vi "2_ExportDatatoExcel.vi"(8 "error in (no error)":errorcluster, 10 "Waveform Graph":waveform(dbl)[](graph), 11 "file path (IN)":path) -> (0 "error out":errorcluster, 3 "file path (OUT)":path)   [LabVIEW 2020]
uses:
  <vilib>/Utility/file.llb/Write Delimited Spreadsheet (string).vi
panel:
  out "Ch3 : Y":dbl[](array[numeric])
  out "Ch3 : appended array":string[](array[string])
  out "Ch2 : Y":dbl[](array[numeric])
  out "Ch2 : appended array":string[](array[string])
  out "Ch1 : appended array":string[](array[string])
  out "Ch1 : Y":dbl[](array[numeric])
  out "dt":dbl
  out "Spread Sheet Display":string[][](array[string])
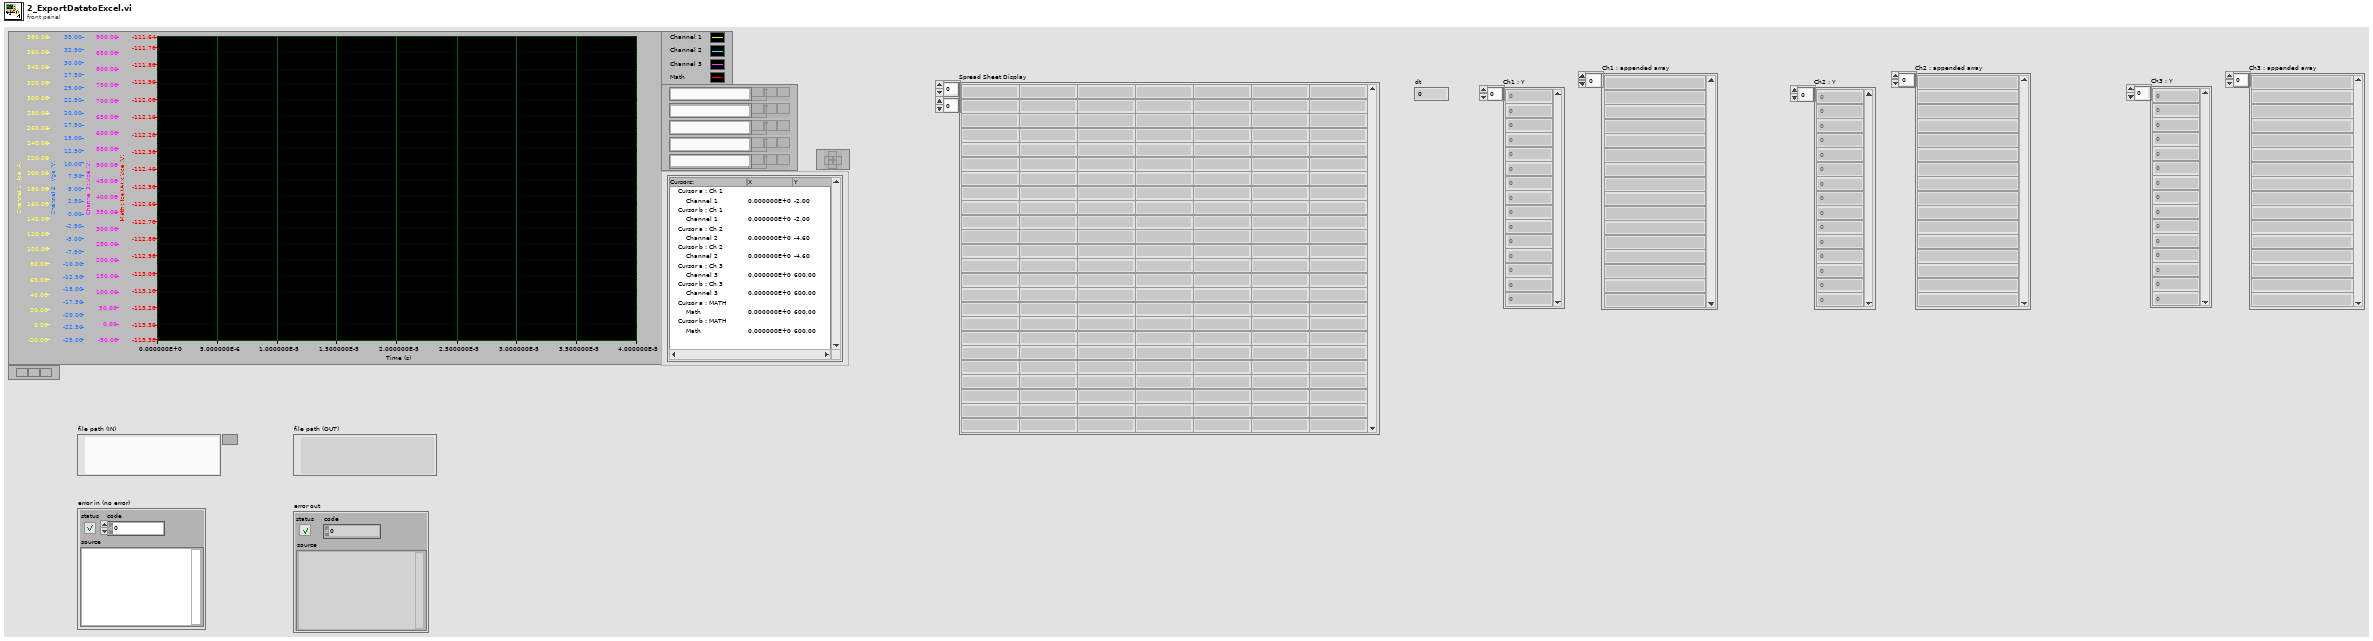
[diagram p1: front panel]
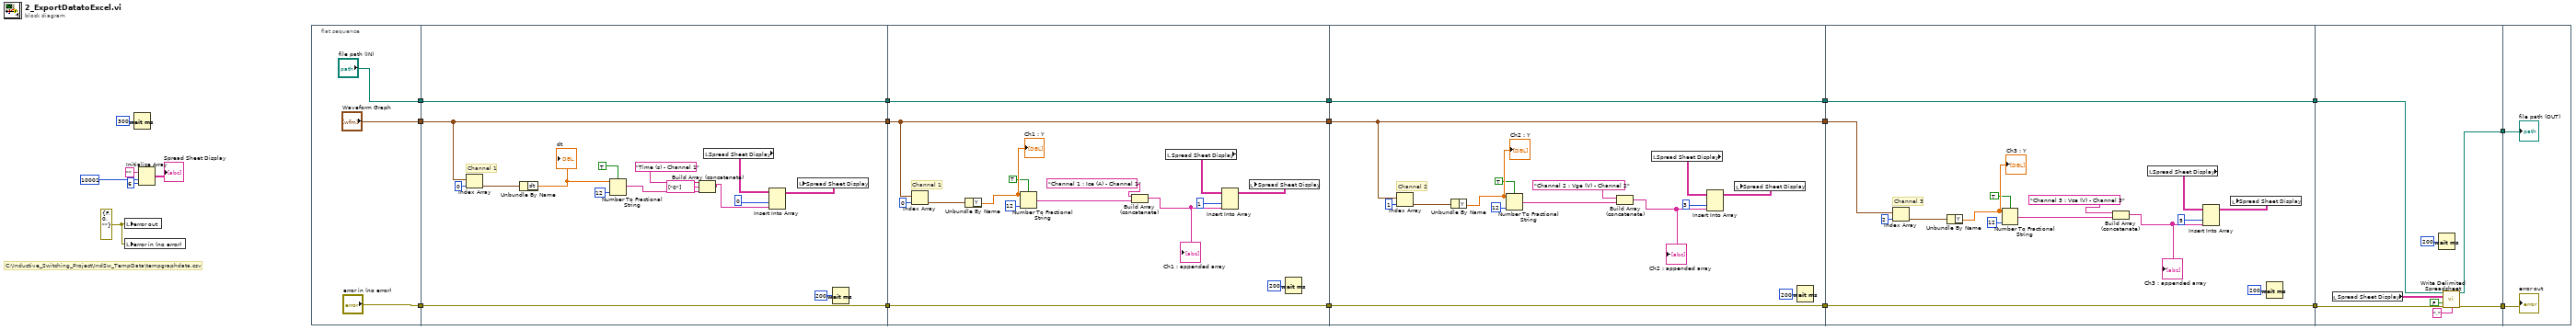
[diagram p0: block diagram]
diagram:
  w7 = errorcluster {"status"=FALSE, "code"=0, "source"=""} ("error out")
  # "C:\\Inductive_Switching_Project\\IndSw_TempData\\tempgraphdata.csv"
  n1 = local write "error out"(w7) -> ()
  n2 = local write "error in (no error)"(w7) -> ()
  n3 = Wait (ms)(milliseconds to wait=u32 300) -> ()  [unwired: 1 out]
  n4 = Initialize Array("", 10001 ("dimension size"), 6 ("dimension size")) -> (→"Spread Sheet Display":string[][])
  n5 = flat-sequence {
    tunnel: ["Waveform Graph"] -> w13
    tunnel: ["error in (no error)"] -> w9
    tunnel: ["file path (IN)"] -> w2
    tunnel: [w29] -> w17
    tunnel: w13 -> [w29]
    tunnel: w9 -> [w28]
    tunnel: [w28] -> w8
    tunnel: [w26] -> w3
    tunnel: w2 -> [w26]
    tunnel: w17 -> [w45]
    tunnel: [w45] -> w16
    tunnel: [w44] -> w10
    tunnel: w8 -> [w44]
    tunnel: [w42] -> w4
    tunnel: w3 -> [w42]
    tunnel: w16 -> [w60]
    tunnel: [w60] -> w15
    tunnel: [w59] -> w11
    tunnel: w10 -> [w59]
    tunnel: [w57] -> w5
    tunnel: w4 -> [w57]
    tunnel: w15 -> [w75]
    tunnel: [w74] -> w12
    tunnel: w11 -> [w74]
    tunnel: [w72] -> w6
    tunnel: w5 -> [w72]
    tunnel: [w91] -> w14
    tunnel: w12 -> [w90]
    tunnel: w6 -> [w88]
    tunnel: [w87] -> w1
    tunnel: w14 -> [w96]
    tunnel: w1 -> [w95]
    frame #0 {
    }
    frame #1 {
      # "Channel 1"
      n6 = Index Array(array=w29, index=0) -> (element=w40:waveform(dbl))
      n7 = Unbundle By Name(w40) -> ("dt"=w38:dbl)
      "dt" <- w38
      n8 = Number To Fractional String(use system decimal point (T)=TRUE, number=w38, precision (6)=i16 12) -> (F-format string=w33:string)  [unwired: 1 in]
      n9 = Build Array (concatenate)("Time (s) - Channel 1", string[] ["0"] ("array"), w33) -> (w32:string[])
      n10 = local read "Spread Sheet Display"() -> (w37:string[][])
      n11 = Insert Into Array(array=w37, index (col)=0 ("disabled index (col)"), new element=w32) -> (w41:string[][])  [unwired: 1 in]
      n12 = local write "Spread Sheet Display"(w41) -> ()
      n13 = Wait (ms)(milliseconds to wait=u32 200) -> ()  [unwired: 1 out]
    }
    frame #2 {
      # "Channel 1"
      n14 = Index Array(array=w45, index=0) -> (element=w52:waveform(dbl))
      n15 = Unbundle By Name(w52) -> ("Y"=w53:dbl[])
      "Ch1 : Y" <- w53
      n16 = Number To Fractional String(use system decimal point (T)=TRUE, number=w53, precision (6)=i16 12) -> (F-format string=w55:string[])  [unwired: 1 in]
      n17 = Build Array (concatenate)("Channel 1 : Ice (A) - Channel 1", w55) -> (w56:string[])
      "Ch1 : appended array" <- w56
      n18 = local read "Spread Sheet Display"() -> (w54:string[][])
      n19 = Insert Into Array(array=w54, index (col)=1 ("disabled index (col)"), new element=w56) -> (w51:string[][])  [unwired: 1 in]
      n20 = local write "Spread Sheet Display"(w51) -> ()
      n21 = Wait (ms)(milliseconds to wait=u32 200) -> ()  [unwired: 1 out]
    }
    frame #3 {
      # "Channel 2"
      n22 = Index Array(array=w60, index=1) -> (element=w71:waveform(dbl))
      n23 = Unbundle By Name(w71) -> ("Y"=w70:dbl[])
      "Ch2 : Y" <- w70
      n24 = Number To Fractional String(use system decimal point (T)=TRUE, number=w70, precision (6)=i16 12) -> (F-format string=w68:string[])  [unwired: 1 in]
      n25 = Build Array (concatenate)("Channel 2 : Vge (V) - Channel 2", w68) -> (w67:string[])
      "Ch2 : appended array" <- w67
      n26 = local read "Spread Sheet Display"() -> (w69:string[][])
      n27 = Insert Into Array(array=w69, index (col)=3 ("disabled index (col)"), new element=w67) -> (w66:string[][])  [unwired: 1 in]
      n28 = local write "Spread Sheet Display"(w66) -> ()
      n29 = Wait (ms)(milliseconds to wait=u32 200) -> ()  [unwired: 1 out]
    }
    frame #4 {
      # "Channel 3"
      n30 = Index Array(array=w75, index=2) -> (element=w82:waveform(dbl))
      n31 = Unbundle By Name(w82) -> ("Y"=w83:dbl[])
      "Ch3 : Y" <- w83
      n32 = Number To Fractional String(use system decimal point (T)=TRUE, number=w83, precision (6)=i16 12) -> (F-format string=w85:string[])  [unwired: 1 in]
      n33 = Build Array (concatenate)("Channel 3 : Vce (V) - Channel 3", w85) -> (w86:string[])
      "Ch3 : appended array" <- w86
      n34 = local read "Spread Sheet Display"() -> (w84:string[][])
      n35 = Insert Into Array(array=w84, index (col)=5 ("disabled index (col)"), new element=w86) -> (w81:string[][])  [unwired: 1 in]
      n36 = local write "Spread Sheet Display"(w81) -> ()
      n37 = Wait (ms)(milliseconds to wait=u32 200) -> ()  [unwired: 1 out]
    }
    frame #5 {
      n38 = local read "Spread Sheet Display"() -> (w94:string[][])
      n39 = Wait (ms)(milliseconds to wait=u32 200) -> ()  [unwired: 1 out]
      n40 = call-poly <vilib>:"Write Delimited Spreadsheet.vi"("file path (dialog if empty)"=w88, "2D data"=w94, "append to file? (new file:F)"=FALSE, "error in (no error)"=w90, "delimiter (\\t)"="," ("delimiter (\\t)")) -> ("new file path (Not A Path if cancelled)"=w87:path, "error out"=w91:errorcluster)  [unwired: 9 in]
    }
    frame #6 {
      "error out" <- w96
      "file path (OUT)" <- w95
    }
  }
